vi "Set Many Attributes Priv.vi"(0 "Tree Dictionary Out":variant, 5 "Unique ID":string, 7 "Name":string[](array[string]), 9 "Data":variant[](array[variant]), 11 "error in":errorcluster) -> (4 "Tree Dictionary Out":variant, 8 "Replaced?":bool[](array[boolean]), 15 "error out":errorcluster)   [LabVIEW 2017, in "Tree API.lvlib" / "Tree.lvclass"]
uses:
  Tree.lvclass
  Typedefs/Tree Cluster.ctl
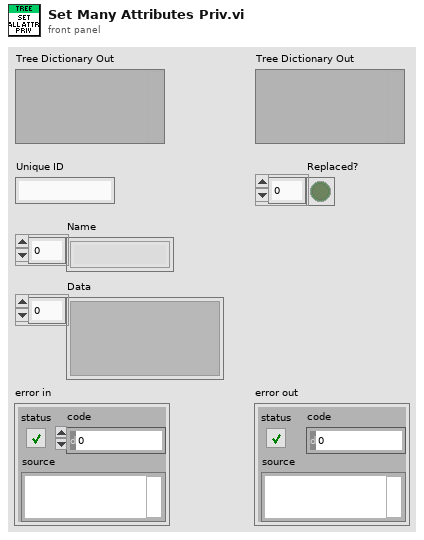
[diagram p1: front panel]
types:
  T1 = typedef "Tree API.lvlib/Tree.lvclass/Tree Cluster.ctl" = cluster{"Unique ID":string, "Parent ID":string, "Child IDs":string[], "Name":string, "MetaData":string, "Data IDs":string[]}
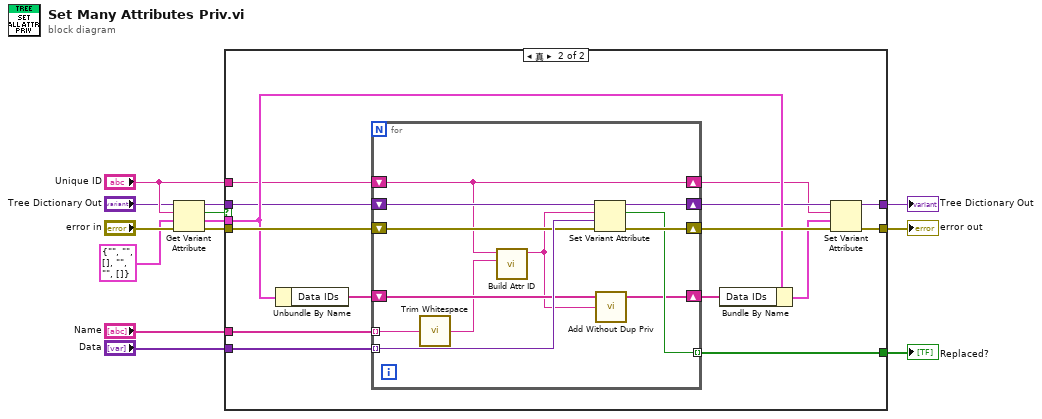
[diagram p0: block diagram]
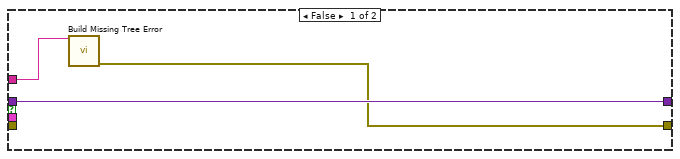
[diagram p2: hidden frame]
diagram:
  n1 = Get Variant Attribute(Variant="Tree Dictionary Out", name="Unique ID", default value (empty Variant)=T1 {"Unique ID"="", "Parent ID"="", "Child IDs"=[], "Name"="", "MetaData"="", "Data IDs"=[]} ("Cluster of class private data"), error in="error in") -> (duplicate Variant=w9:variant, found=w10:bool, value=w11:T1, error out=w7:errorcluster)
  n2 = case shown="真" w10 {
    tunnel: [w14 w31] -> w5
    tunnel: [w16 w30] -> w6
    tunnel: w7 -> [_ w28]
    tunnel: w9 -> [w16 w21]
    tunnel: w11 -> [_ w26]
    tunnel: "Name" -> [_ w23]
    tunnel: "Data" -> [_ w29]
    tunnel: "Unique ID" -> [w15 w20]
    tunnel: [_ w24] -> w3
    frame False {
      n3 = call "Build Missing Tree Error.vi"("Unique ID"=w15) -> ("Error Out"=w14:errorcluster)  [unwired: 14 in]
    }
    frame True {
      n4 = Unbundle By Name(w26) -> ("Data IDs"=w18:string[])
      n5 = for {
        tunnel: w29 -> [w42] mode=indexing
        tunnel: w23 -> [w36] mode=indexing
        tunnel: [w38] -> w24 mode=indexing
        shift-right: [w40] -> w27
        shift-left: w28 -> [w41]
        shift-right: [w43] -> w22
        shift-left: w21 -> [w39]
        shift-right: [w37] -> w19
        shift-left: w20 -> [w37]
        shift-right: [w33] -> w17
        shift-left: w18 -> [w35]
        n6 = call <vilib>:"Trim Whitespace.vi"("string"=w36) -> ("trimmed string"=w32:string)  [unwired: 1 in]
        n7 = call "Build Attr ID.vi"("Attr Name"=w32, "Unique ID"=w37) -> ("Attr ID Out"=w34:string)  [unwired: 9 in]
        n8 = Set Variant Attribute(Variant=w39, name=w34, value=w42, error in=w41) -> (Variant out=w43:variant, replaced=w38:bool, error out=w40:errorcluster)
        n9 = call "Add Without Dup Priv.vi"("Add String"=w34, "Strings In"=w35) -> ("Strings Out"=w33:string[])  [unwired: 3 in]
      }
      n10 = Bundle By Name(cluster=w26, "Data IDs"=w17) -> (w25:T1)
      n11 = Set Variant Attribute(Variant=w22, name=w19, value=w25, error in=w27) -> (Variant out=w30:variant, error out=w31:errorcluster)  [unwired: 1 out]
    }
  }
  "Tree Dictionary Out" <- w6
  "error out" <- w5
  "Replaced?" <- w3
